vi "RaFMenuFixer.vi"(6 "Tableau des filtres":string[](array[string]), 11 "Prefix":string) -> (5 "Item Tags":string[](array[string]), 7 "Item Names":string[](array[string]))   [LabVIEW 2019]
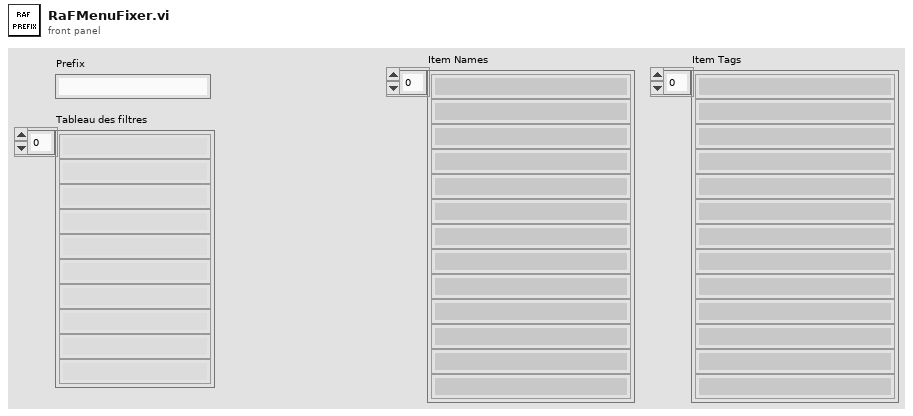
[diagram p1: front panel]
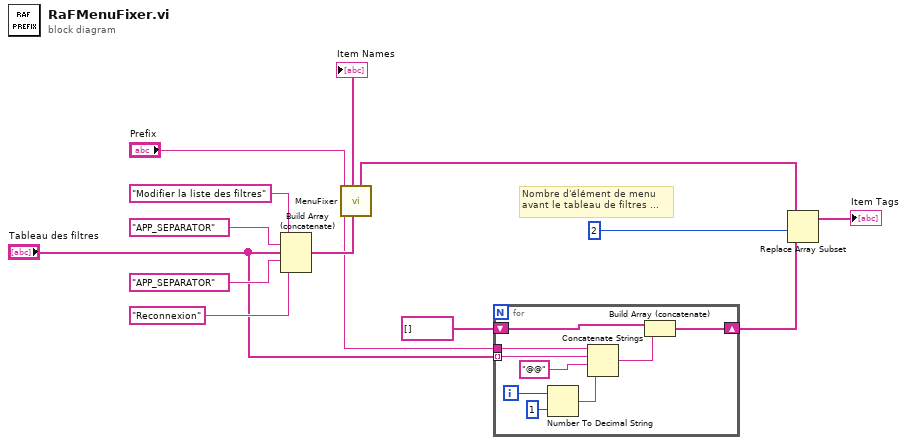
[diagram p0: block diagram]
diagram:
  # "Nombre d'élément de menu\navant le tableau de filtres ..."
  n1 = Build Array (concatenate)("Modifier la liste des filtres" ("menu tag"), "APP_SEPARATOR" ("menu tag"), "Tableau des filtres", "APP_SEPARATOR" ("menu tag"), "Reconnexion" ("menu tag")) -> (w8:string[])
  n2 = call "MenuFixer.vi"("Menu Name"=w8, "Prefix"="Prefix") -> ("Item Tags"=w5:string[], "Item Names"=→"Item Names":string[])  [unwired: 8 in]
  n3 = for {
    shift-right: [w21] -> w4
    shift-left: string[] [] -> [w22]
    tunnel: "Tableau des filtres" -> [w19] mode=indexing
    tunnel: "Prefix" -> [w14]
    i -> [w20]
    n4 = Number To Decimal String(number=w20, width (-)=i16 1) -> (decimal integer string=w16:string)
    n5 = Concatenate Strings(w14, w19, "@@" ("string"), w16) -> (w17:string)
    n6 = Build Array (concatenate)(w22, w17) -> (w21:string[])
  }
  n7 = Replace Array Subset(array=w5, new element=w4, index=2) -> (→"Item Tags":string[])
